vi "Get best DAQ settings.vi"(7 "Sine waves to average":i32=1, 8 "Slowest acceptable update interval, s":dbl=0.25, 9 "Optimal number of samples per read":i32=20000, 10 "Samples per sine wave":i32=100, 11 "Sine frequency, Hz":dbl=1000.0 format="%#_6p") -> (3 "Samples per read":i32)   [LabVIEW 2020]
doc: "Determine how many samples read at once in multiples of sine waves to average. Optimize number of samples per read for faster data throughput, but not longer than a slowest interval."
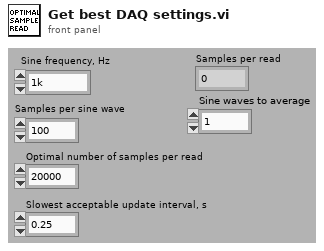
[diagram p1: front panel]
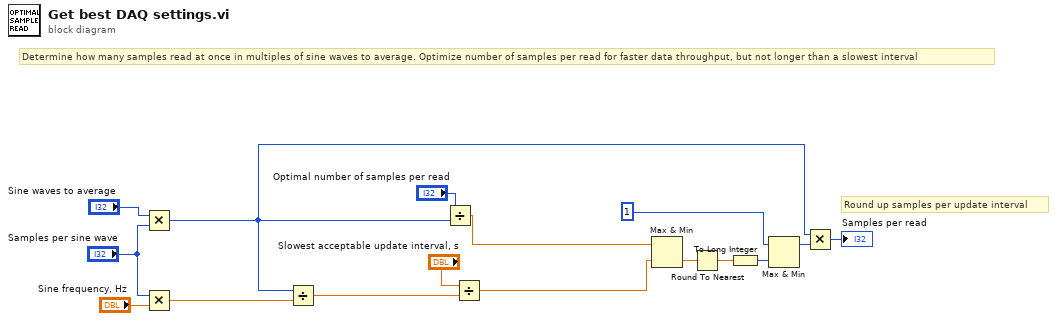
[diagram p0: block diagram]
diagram:
  # "Determine how many samples read at once in multiples of sine waves to average. Optimize number of samples per read for faster data throughput, but not longer than a slowest interval"
  # "Round up samples per update interval"
  n1 = Multiply(x="Sine waves to average", y="Samples per sine wave") -> (x*y=w8:i32)
  n2 = Multiply(x="Samples per sine wave", y="Sine frequency, Hz") -> (x*y=w7:dbl)
  n3 = Divide(x=w8, y=w7) -> (x/y=w5:dbl)
  n4 = Divide(x="Optimal number of samples per read", y=w8) -> (x/y=w15:dbl)
  n5 = Divide(x="Slowest acceptable update interval, s", y=w5) -> (x/y=w4:dbl)
  n6 = Max & Min(x=w15, y=w4) -> (min(x,y)=w3:dbl)  [unwired: 1 out]
  n7 = Round To Nearest(number=w3) -> (nearest integer value=w14:dbl)
  n8 = To Long Integer(number=w14) -> (32bit integer=w12:i32)
  n9 = Max & Min(x=1, y=w12) -> (max(x,y)=w10:i32)  [unwired: 1 out]
  n10 = Multiply(x=w8, y=w10) -> (x*y=→"Samples per read":i32)
